vi "Read_JT.vi"(2 "error in":errorcluster, 3 "Write":string, 4 "connection ID":refnum<k5>) -> (0 "error out":errorcluster, 1 "Read":string)   [LabVIEW 2016]
uses:
  Instrument_Setup.vi
panel:
  out "String":string
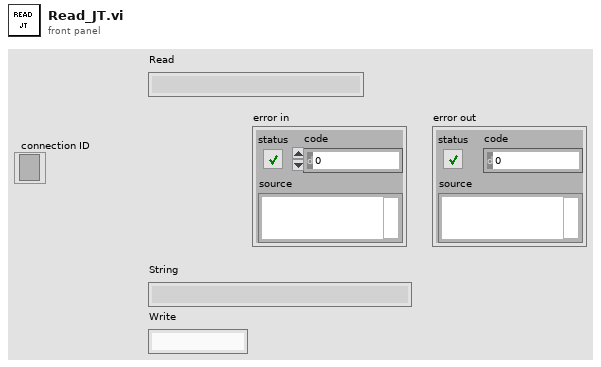
[diagram p1: front panel]
types:
  T1 = cluster{"Mode":enum16{"Standard", "Buffered", "CRLF", "Immediate"}, "Bytes to Read":i32, "IP Address":string, "Remote Port":i32, "Timeout":i32}
  T2 = enum16{"Standard", "Buffered", "CRLF", "Immediate"}
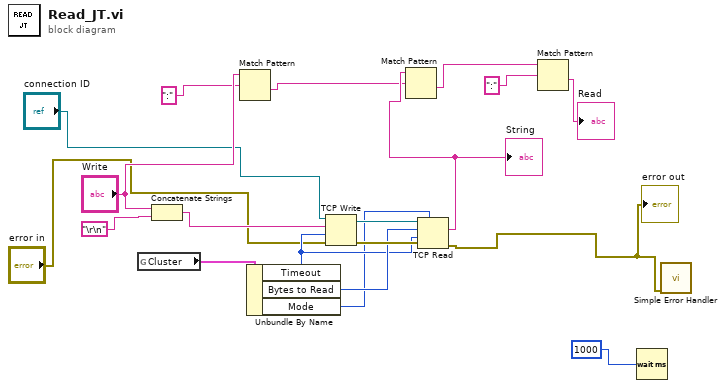
[diagram p0: block diagram]
diagram:
  n1 = global read "Instrument_Setup.vi" "Cluster"() -> (w18:T1)
  n2 = Concatenate Strings("Write", "\r\n") -> (w11:string)
  n3 = Match Pattern(string="Write", regular expression=":") -> (after substring=w8:string)  [unwired: 1 in, 3 out]
  n4 = Unbundle By Name(w18) -> ("Timeout"=w15:i32, "Bytes to Read"=w16:i32, "Mode"=w14:T2)
  n5 = TCP Write(connection ID="connection ID", data in=w11, error in (no error)="error in", 9:w15) -> (connection ID out=w19:refnum<k5>, error out=w17:errorcluster)  [unwired: 1 out]
  n6 = TCP Read(connection ID=w19, bytes to read=w16, error in (no error)=w17, 7:w14, 9:w15) -> (data out=w12:string, error out=w1:errorcluster)  [unwired: 1 out]
  "String" <- w12
  "error out" <- w1
  n7 = Match Pattern(string=w12, regular expression=w8) -> (after substring=w5:string)  [unwired: 1 in, 3 out]
  n8 = Match Pattern(string=w5, regular expression=":") -> (after substring=→"Read":string)  [unwired: 1 in, 3 out]
  n9 = Wait (ms)(milliseconds to wait=1000) -> ()  [unwired: 1 out]
  n10 = call <vilib>:"Simple Error Handler.vi"("error in (no error)"=w1) -> ()  [unwired: 4 in, 5 out]
